vi "destroyEvents.vi"(8 "error in (no error)":errorcluster, 11 "PubSubDataEvent in":refnum<class "PubSubDataEvent.lvclass">) -> (0 "error out":errorcluster, 3 "PubSubDataEvent out":refnum<class "PubSubDataEvent.lvclass">)   [LabVIEW 2016, in "PubSubDataEvent.lvclass"]
uses:
  PubSubDataEvent.lvclass
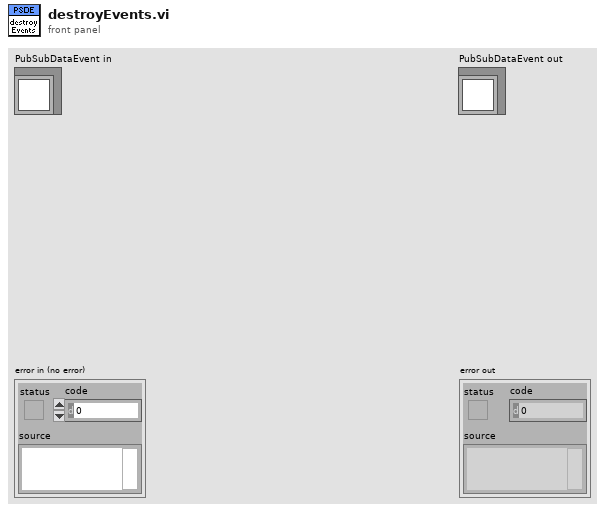
[diagram p1: front panel]
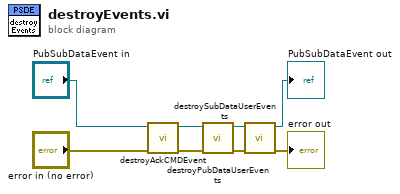
[diagram p0: block diagram]
diagram:
  n1 = call "destroyAckCMDEvent.vi"("error in (no error)"="error in (no error)", "PubSubDataEvent in"="PubSubDataEvent in") -> ("error out"=w4:errorcluster, "PubSubDataEvent out"=w1:refnum<class "PubSubDataEvent.lvclass">)  [unwired: 8 in]
  n2 = call "destroyPubDataUserEvents.vi"("error in (no error)"=w4, "PubSubDataEvent in"=w1) -> ("error out"=w6:errorcluster, "PubSubDataEvent out"=w8:refnum<class "PubSubDataEvent.lvclass">)  [unwired: 8 in]
  n3 = call "destroySubDataUserEvents.vi"("error in (no error)"=w6, "PubSubDataEvent in"=w8) -> ("error out"=→"error out":errorcluster, "PubSubDataEvent out"=→"PubSubDataEvent out":refnum<class "PubSubDataEvent.lvclass">)  [unwired: 8 in]
